vi "Generate Report.vi"(8 "error in (no error)":errorcluster, 11 "Web Reports in":refnum<class "Web Reports.lvclass">) -> (0 "error out":errorcluster, 3 "Web Reports out":refnum<class "Web Reports.lvclass">)   [LabVIEW 2020, in "Web Reports.lvclass"]
uses:
  Web Reports.lvclass
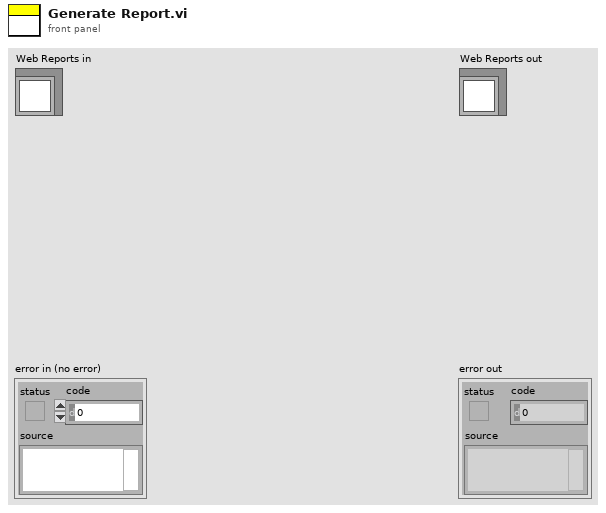
[diagram p1: front panel]
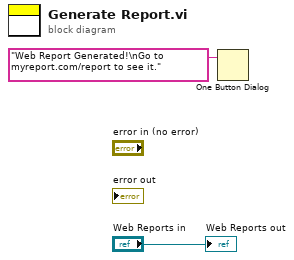
[diagram p0: block diagram]
diagram:
  n1 = One Button Dialog(message="Web Report Generated!\nGo to myreport.com/report to see it.") -> ()  [unwired: 1 in, 1 out]
  "Web Reports out" <- "Web Reports in"
